vi "Measure.vi"(0 "NI-DMM in":refnum<class "NI-DMM.lvclass">, 5 "Measure_Parameters":variant, 11 "error in (no error)":errorcluster) -> (4 "NI-DMM out":refnum<class "NI-DMM.lvclass">, 6 "Measure_Results":variant, 15 "error out":errorcluster)   [LabVIEW 2020, in "Abstract_Instrument.lvlib" / "NI-DMM.lvclass"]
uses:
  NI-DMM.lvclass
  <vilib>/MeasurementLink/MeasurementLink niDMM/MeasurementLink niDMM.lvlib
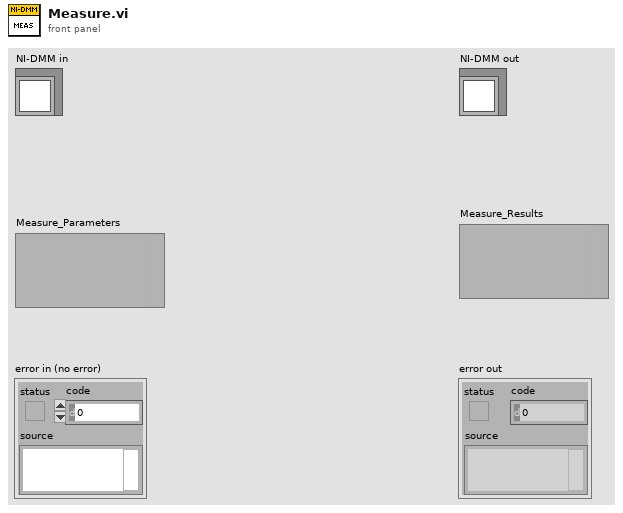
[diagram p1: front panel]
types:
  T1 = typedef "MeasurementLink niDMM.lvlib/Connection with Session.ctl" = cluster{"connection":T2, "session":refnum<k15>}
  T2 = typedef "MeasurementLink Session Management V1.lvlib/Session Reservation.lvclass/Connection.ctl" = cluster{"pin or relay name":string, "site":i32, "instrument type id":string, "channel":string}
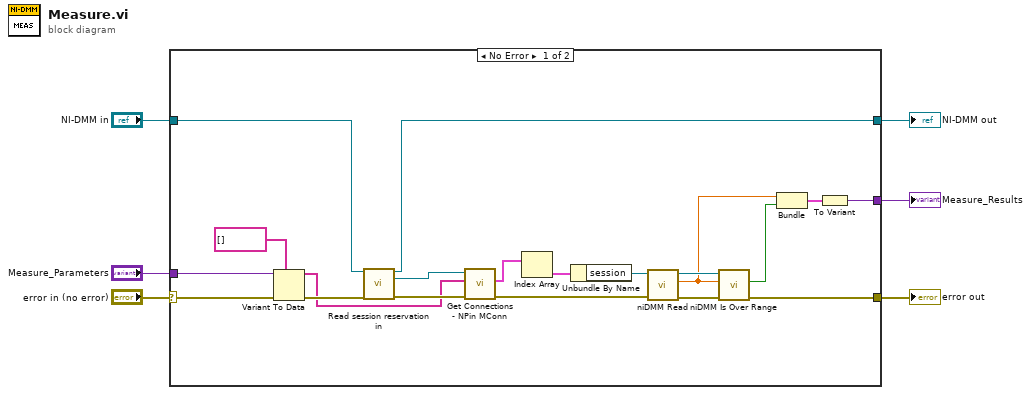
[diagram p0: block diagram]
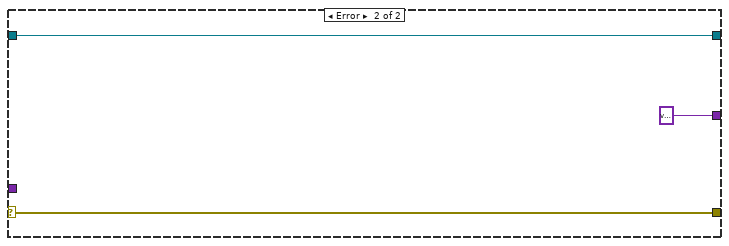
[diagram p2: hidden frame]
diagram:
  n1 = case shown="No Error" "error in (no error)" {
    selector: "error in (no error)" -> [w18 w27]
    tunnel: [w25 w27] -> w5
    tunnel: "NI-DMM in" -> [w11 w29]
    tunnel: [w20 variant ("Variant")] -> w3
    tunnel: [w12 w29] -> w2
    tunnel: "Measure_Parameters" -> [w17 _]
    frame No Error {
      n2 = Variant To Data(error in=w18, type=string[] [], Variant=w17) -> (data=w10:string[], error out=w15:errorcluster)
      n3 = call-dynamic "Read session reservation in.vi"("AbstractDMM in"=w11, "error in (no error)"=w15) -> ("AbstractDMM out"=w12:refnum<class "NI-DMM.lvclass">, "MeasurementLink Session Management V1.lvlib:Session Reservation.lvclass"=w16:refnum<class "Session Reservation.lvclass">, "error out"=w14:errorcluster)  [unwired: 11 in]
      n4 = call <vilib>:"Get Connections - NPin MConn.vi"("error in"=w14, "pin or relay names"=w10, "session reservation in"=w16) -> ("error out"=w13:errorcluster, "connections"=w9:T1[])  [unwired: 6 in, 1 out]
      n5 = Index Array(array=w9) -> (element=w8:T1)  [unwired: 1 in]
      n6 = Unbundle By Name(w8) -> ("session"=w7:refnum<k15>)
      n7 = call <instrlib>:"niDMM Read.vi"("error in (no error)"=w13, "instrument handle"=w7) -> ("error out"=w26:errorcluster, "Measurement"=w23:dbl, "instrument handle out"=w24:refnum<k15>)  [unwired: 7 in]
      n8 = call <instrlib>:"niDMM Is Over Range.vi"("error in (no error)"=w26, "Measurement"=w23, "instrument handle"=w24) -> ("error out"=w25:errorcluster, "Over Range?"=w22:bool)  [unwired: 6 in, 1 out]
      n9 = Bundle("Measurement"=w23, "Over Range?"=w22) -> (w21:cluster{"Measurement":dbl, "Over Range?":bool})  [unwired: 1 in]
      n10 = To Variant(anything=w21) -> (Variant=w20:variant)
    }
    frame Error {
    }
  }
  "error out" <- w5
  "NI-DMM out" <- w2
  "Measure_Results" <- w3
